vi "CheckForDevices.vi"(6 "error in":errorcluster) -> (0 "error out":errorcluster, 2 "Device Types":string[](array[string]), 3 "Device Handles":u64[](array[numeric]))   [LabVIEW 2023, in "Coherent Laser.lvlib"]
uses:
  Coherent Laser.lvlib
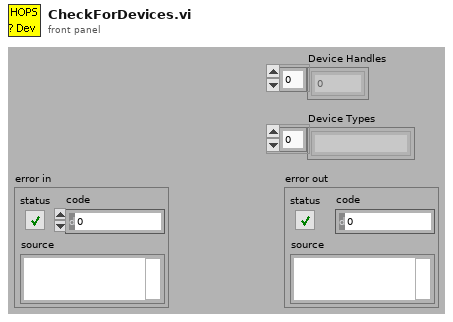
[diagram p1: front panel]
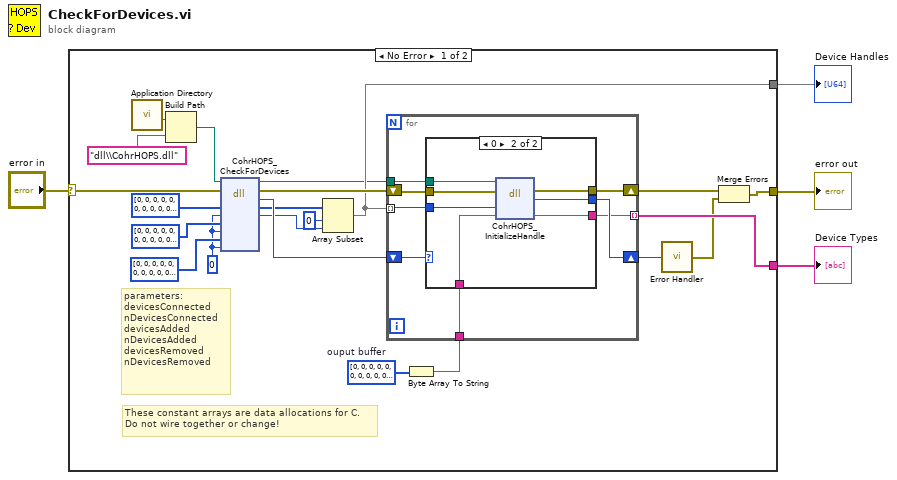
[diagram p0: block diagram]
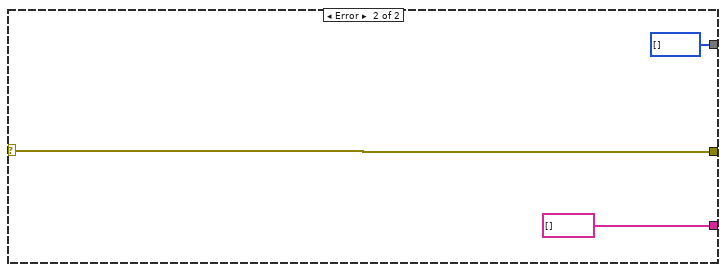
[diagram p3: hidden frame]
diagram:
  n1 = case shown="No Error" "error in" {
    selector: "error in" -> [w16 w45]
    tunnel: [w17 w45] -> w4
    tunnel: [w20 string[] []] -> w3
    tunnel: [w11 u64[] []] -> w1
    frame No Error {
      w10 = u8[] [0, 0, 0, 0, 0, 0, 0, 0, 0, 0, 0, 0, 0, 0, 0, 0, 0, 0, 0, 0, 0, 0, 0, 0, 0, 0, 0, 0, 0, 0, 0, 0, 0, 0, 0, 0, 0, 0, 0, 0, 0, 0, 0, 0, 0, 0, 0, 0, 0, 0, 0, 0, 0, 0, 0, 0, 0, 0, 0, 0, 0, 0, 0, 0, 0, 0, 0, 0, 0, 0, 0, 0, 0, 0, 0, 0, 0, 0, 0, 0, 0, 0, 0, 0, 0, 0, 0, 0, 0, 0, 0, 0, 0, 0, 0, 0, 0, 0, 0, 0, 1]  # ouput buffer
      w22 = u64 0 ("Input Value")
      # "These constant arrays are data allocations for C.\nDo not wire together or change!"
      # "parameters:\ndevicesConnected\nnDevicesConnected\ndevicesAdded\nnDevicesAdded\ndevicesRemoved\nnDevicesRemoved"
      n2 = call <vilib>:"Application Directory.vi"() -> ("Application Directory"=w8:path)
      n3 = Build Path(base path=w8, name or relative path="dll\\CohrHOPS.dll") -> (appended path=w6:path)
      n4 = dll-call lib="?" fn="CohrHOPS_CheckForDevices" label="CheckForDevices"(path in=w6, error in=w16, "arg1"=u64[] [0, 0, 0, 0, 0, 0, 0, 0, 0, 0, 0, 0, 0, 0, 0, 0, 0, 0, 0, 0, 0, 0, 0, 0, 0, 0, 0, 0, 0, 0, 0, 0, 0, 0, 0, 0, 0, 0, 0, 0, 0, 0, 0, 0, 0, 0, 0, 0, 0, 0, 0, 0, 0, 0, 0, 0, 0, 0, 0, 0, 0, 0, 0, 0, 0, 0, 0, 0, 0, 0, 0, 0, 0, 0, 0, 0, 0, 0, 0, 0, 0, 0, 0, 0, 0, 0, 0, 0, 0, 0, 0, 0, 0, 0, 0, 0, 0, 0, 0, 0, 1] ("devicesRemoved"), "arg2"=w22, "arg3"=u64[] [0, 0, 0, 0, 0, 0, 0, 0, 0, 0, 0, 0, 0, 0, 0, 0, 0, 0, 0, 0, 0, 0, 0, 0, 0, 0, 0, 0, 0, 0, 0, 0, 0, 0, 0, 0, 0, 0, 0, 0, 0, 0, 0, 0, 0, 0, 0, 0, 0, 0, 0, 0, 0, 0, 0, 0, 0, 0, 0, 0, 0, 0, 0, 0, 0, 0, 0, 0, 0, 0, 0, 0, 0, 0, 0, 0, 0, 0, 0, 0, 0, 0, 0, 0, 0, 0, 0, 0, 0, 0, 0, 0, 0, 0, 0, 0, 0, 0, 0, 0, 1] ("devicesRemoved"), "arg4"=w22, "arg5"=u64[] [0, 0, 0, 0, 0, 0, 0, 0, 0, 0, 0, 0, 0, 0, 0, 0, 0, 0, 0, 0, 0, 0, 0, 0, 0, 0, 0, 0, 0, 0, 0, 0, 0, 0, 0, 0, 0, 0, 0, 0, 0, 0, 0, 0, 0, 0, 0, 0, 0, 0, 0, 0, 0, 0, 0, 0, 0, 0, 0, 0, 0, 0, 0, 0, 0, 0, 0, 0, 0, 0, 0, 0, 0, 0, 0, 0, 0, 0, 0, 0, 0, 0, 0, 0, 0, 0, 0, 0, 0, 0, 0, 0, 0, 0, 0, 0, 0, 0, 0, 0, 1] ("devicesRemoved"), "arg6"=w22) -> (path out=w5:path, error out=w25:errorcluster, "return type"=w15:i32, "arg1"=w14:u64[], "arg2"=w13:u64)  [unwired: 5 in]
      n5 = Array Subset(array=w14, index=0, length=w13) -> (w11:u64[])
      n6 = Byte Array To String(unsigned byte array=w10) -> (string=w9:string)
      n7 = for {
        shift-right: [w34] -> w26
        shift-left: w15 -> [w29]
        tunnel: w11 -> [w33] mode=indexing
        tunnel: [w32] -> w20 mode=indexing
        shift-right: [w30] -> w19
        shift-left: w25 -> [w31]
        tunnel: w9 -> [w28]
        tunnel: w5 -> [w27]
        n8 = case shown="0" w29 {
          selector: w29 -> [w36 _]
          tunnel: [w36 w44] -> w34
          tunnel: w33 -> [_ w43]
          tunnel: ["" w42] -> w32
          tunnel: w31 -> [w35 w41]
          tunnel: [w35 w40] -> w30
          tunnel: w28 -> [_ w39]
          tunnel: w27 -> [_ w38]
          frame Default {
            (unwired) -1 ("index of element")
            # "an error has occurred"
          }
          frame 0 {
            n9 = dll-call lib="?" fn="CohrHOPS_InitializeHandle" label="InitializeHandle"(path in=w38, error in=w41, "arg1"=w43, "arg2"=w39) -> (error out=w40:errorcluster, "return type"=w44:i32, "arg2"=w42:string)  [unwired: 2 in, 1 out]
          }
        }
      }
      n10 = call "Error Handler.vi"("Return Value"=w26) -> ("error out"=w18:errorcluster)
      n11 = Merge Errors(w19, w18) -> (w17:errorcluster)
    }
    frame Error {
    }
  }
  "error out" <- w4
  "Device Types" <- w3
  "Device Handles" <- w1
